vi "05.Evd.2_Ask.5.vi"() -> ()   [LabVIEW 2020]
panel:
  out "Win B":bool
  out "Win A":bool
  out "Tie":bool
  out "B":dbl
  out "A":dbl
  in  "B":dbl
  in  "A":dbl
  in  "Boolean":bool
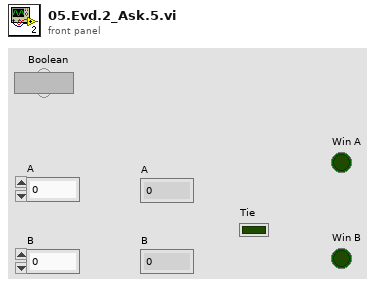
[diagram p1: front panel]
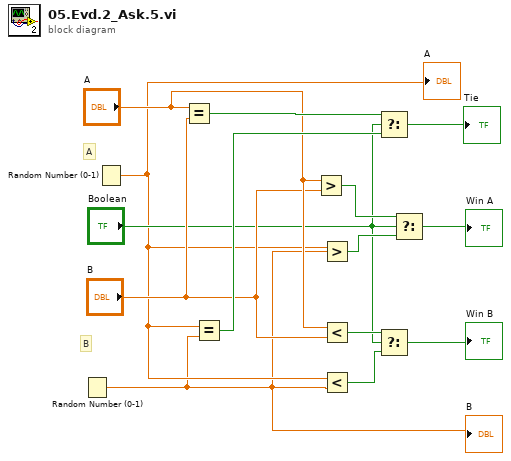
[diagram p0: block diagram]
diagram:
  # "B"
  # "A"
  n1 = Random Number (0-1)() -> (number: 0 to 1=w3:dbl)
  "B" <- w3
  n2 = Random Number (0-1)() -> (number: 0 to 1=w4:dbl)
  "A" <- w4
  n3 = Equal?(x="A", y="B") -> (x = y?=w14:bool)
  n4 = Equal?(x=w4, y=w3) -> (x = y?=w12:bool)
  n5 = Greater?(x="A", y="B") -> (0:w10:bool)
  n6 = Greater?(x=w4, y=w3) -> (0:w9:bool)
  n7 = Less?(x="A", y="B") -> (x < y?=w6:bool)
  n8 = Less?(x=w4, y=w3) -> (x < y?=w2:bool)
  n9 = Select(t=w14, s="Boolean", f=w12) -> (s? t:f=→"Tie":bool)
  n10 = Select(t=w6, s="Boolean", f=w2) -> (s? t:f=→"Win B":bool)
  n11 = Select(t=w10, s="Boolean", f=w9) -> (s? t:f=→"Win A":bool)
